vi "udateSuccesfulTimer.vi"(8 "error in (no error)":errorcluster, 11 "MonoHeartbeat in":refnum<class "MonoHeartbeat.lvclass">) -> (0 "error out":errorcluster, 3 "MonoHeartbeat out":refnum<class "MonoHeartbeat.lvclass">)   [LabVIEW 2016, in "MonoHeartbeat.lvclass"]
uses:
  MonoHeartbeat.lvclass
  MonoHeartbeat.lvclass/MonoHeartbeat.ctl
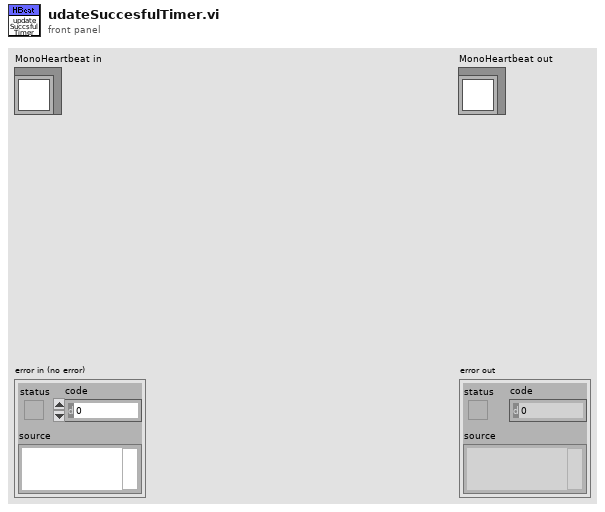
[diagram p1: front panel]
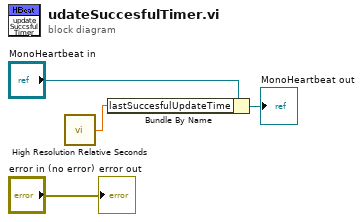
[diagram p0: block diagram]
diagram:
  n1 = call <vilib>:"High Resolution Relative Seconds.vi"() -> ("relative seconds"=w1:dbl)
  n2 = Bundle By Name(cluster="MonoHeartbeat in", "lastSuccesfulUpdateTime"=w1) -> (→"MonoHeartbeat out":refnum<class "MonoHeartbeat.lvclass">)
  "error out" <- "error in (no error)"
